vi "sub_DWA_dwa-control.vi"() -> ()   [LabVIEW 2019]
panel:
  out "dw":dbl[](array[numeric])
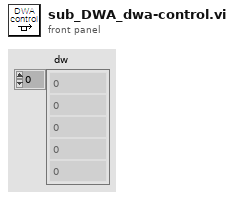
[diagram p1: front panel]
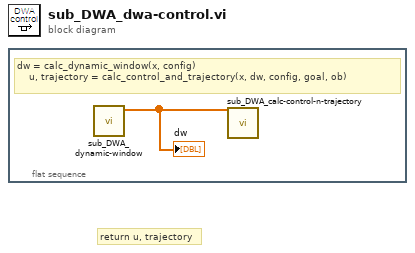
[diagram p0: block diagram]
diagram:
  # "return u, trajectory"
  n1 = flat-sequence {
    frame #0 {
      # "dw = calc_dynamic_window(x, config)\n    u, trajectory = calc_control_and_trajectory(x, dw, config, goal, ob)"
      n2 = call "sub_DWA_dynamic-window.vi"() -> ("dw"=w1:dbl[])  [unwired: 11 in]
      "dw" <- w1
      n3 = call "sub_DWA_calc-control-n-trajectory.vi"("dw"=w1) -> ()  [unwired: 11 in]
    }
  }
